vi "SiftForLine.vi"(9 "Current Line":i32, 11 "All Lines":T2) -> (3 "Line connections":T1[](array[typedef]))   [LabVIEW 2014]
uses:
  Libraries/Map Data Folder/All-Lines.ctl
  Libraries/Map Data Folder/LineCluster.ctl
  Libraries/Map Data Folder/LineConnection.ctl
  Libraries/Map Data Folder/Map Data.lvlib
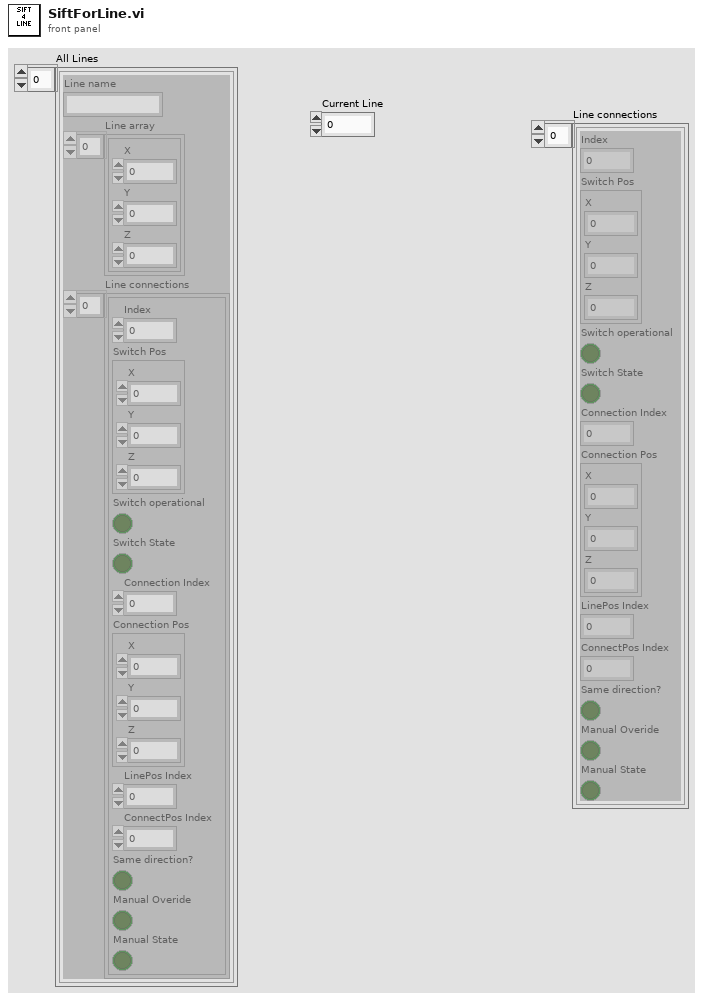
[diagram p1: front panel]
types:
  T1 = typedef "LineConnection.ctl" = cluster{"Index":i32, "Switch Pos":cluster{"X":dbl, "Y":dbl, "Z":dbl}, "Switch operational":bool, "Switch State":bool, "Connection Index":i32, "Connection Pos":cluster{"X":dbl, "Y":dbl, "Z":dbl}, "LinePos Index":i32, "ConnectPos Index":i32, "Same direction?":bool, "Manual Overide":bool, "Manual State":bool}
  T2 = typedef "Map Data.lvlib/All-Lines.ctl" = T3[]
  T3 = typedef "Map Data.lvlib/LineCluster.ctl" = cluster{"Line name":string, "Line array":cluster{"X":dbl, "Y":dbl, "Z":dbl}[], "Line connections":T1[]}
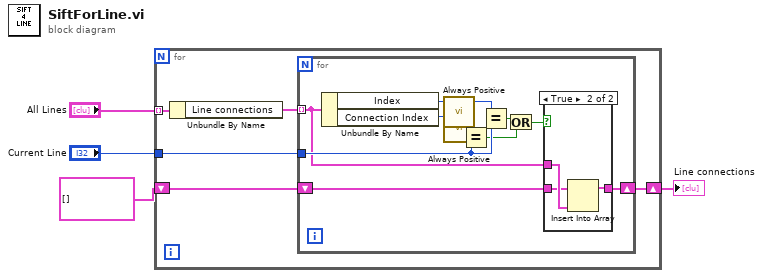
[diagram p0: block diagram]
diagram:
  n1 = for {
    tunnel: "All Lines" -> [w9] mode=indexing
    tunnel: "Current Line" -> [w7]
    shift-right: [w6] -> w1
    shift-left: T1[] [] -> [w5]
    n2 = Unbundle By Name(w9) -> ("Line connections"=w8:T1[])
    n3 = for {
      tunnel: w8 -> [w12] mode=indexing
      tunnel: w7 -> [w16]
      shift-right: [w11] -> w6
      shift-left: w5 -> [w10]
      n4 = Unbundle By Name(w12) -> ("Index"=w19:i32, "Connection Index"=w20:i32)
      n5 = call "Always Positive.vi"("Input"=w19) -> ("Output"=w18:i32)  [unwired: 8 in]
      n6 = call "Always Positive.vi"("Input"=w20) -> ("Output"=w17:i32)  [unwired: 8 in]
      n7 = Equal?(x=w17, y=w16) -> (x = y?=w14:bool)
      n8 = Equal?(x=w18, y=w16) -> (x = y?=w15:bool)
      n9 = Or(x=w15, y=w14) -> (x .or. y?=w13:bool)
      n10 = case shown="True" w13 {
        tunnel: w12 -> [_ w24]
        tunnel: [w21 w23] -> w11
        tunnel: w10 -> [w21 w22]
        frame False {
        }
        frame True {
          n11 = Insert Into Array(array=w22, new element=w24) -> (w23:T1[])  [unwired: 1 in]
        }
      }
    }
  }
  "Line connections" <- w1
